vi "写入固件.vi"(8 "错误输入":errorcluster, 11 "MB session in":refnum<class "MB_Master.lvclass">) -> (0 "error out":errorcluster, 3 "MB session out":refnum<class "MB_Master.lvclass">)   [LabVIEW 2016, in "斯坦道氨氮.lvlib"]
uses:
  <vilib>/Plasmionique/MB Master/MB_Master/MB_Master.lvclass
  <vilib>/NI/Progress Bar/Controls/Update Bar Actions.ctl
  <vilib>/NI/Progress Bar/Controls/Progress Bar Properties.ctl
  <vilib>/Plasmionique/MB Master/MB_Master_Serial/MB_Master_Serial.lvclass
  C:/Program Files (x86)/National Instruments/LabVIEW 2016/vi.lib/Plasmionique/MB Master/MB_Master/MB_Master.lvclass
  <vilib>/Plasmionique/MB Master/MB Master.lvlib
  <vilib>/NI/Progress Bar/Progress Bar.lvlib
panel:
  in  "引用选择":enum16{"MB引用", "自建引用"}(ring)
  in  "VISA Resource":refnum<visa-resource-name>
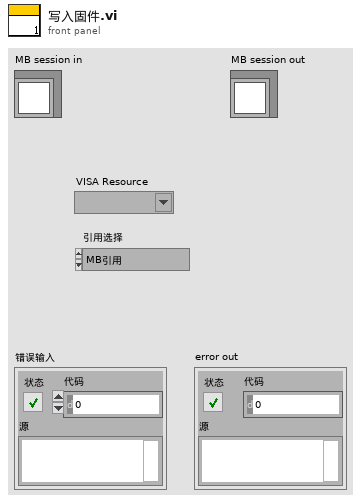
[diagram p1: front panel]
types:
  T1 = enum16{"open", "replace", "create", "open or create", "replace or create", "replace or create with confirmation"}
  T2 = enum16{"big-endian, network order", "native, host order", "little-endian"}
  T3 = typedef "Progress Bar.lvlib/Update Bar Actions.ctl" = enum16{"Add To Existing", "Set to Value"}
  T4 = cluster{"baud rate (bps)":u32, "stop bits":u16, "parity":u16, "flow control":u16, "timeout":u32, "retries":i32}
  T5 = typedef "Progress Bar.lvlib/Progress Bar Properties.ctl" = cluster{"Background Color":u32, "Installer Title":string, "Title Color":u32, "Action Text":string, "Text Color":u32, "Slider Value":u8, "Bar Color":u32, "Timeout":i32}
  T6 = cluster{"泵类型":u8, "进样速度":u32, "出样速度":u32, "泵阀量":u8, "光谱仪类型":u8, "光谱采样次数":u8, "氙灯次数":u8, "B":u16, "C":u16, "D":u16, "E":u16, "B_COD":u16, "C_COD":u16, "D_COD":u16, "E_COD":u16, "G":u16, "M":u16, "N":u16, "氨氮注射泵控温下限":sgl, "氨氮注射泵控温上限":sgl, "总氮注射泵控温下限":sgl, "总氮注射泵控温上限":sgl, "消解温度下限":sgl, "消解温度上限":sgl, "加热10s限值":sgl, "高温高压阀开阀温度":sgl, "总氮x公式0":u8, "总氮x公式1":sgl, "总氮x公式2":sgl, "总磷浊度稀释系数":sgl, "总磷浊度补偿权重1":sgl, "总磷浊度补偿权重2":sgl, "盐度系数":sgl, "氨氮补偿系数1":sgl, "氨氮补偿系数2":sgl}
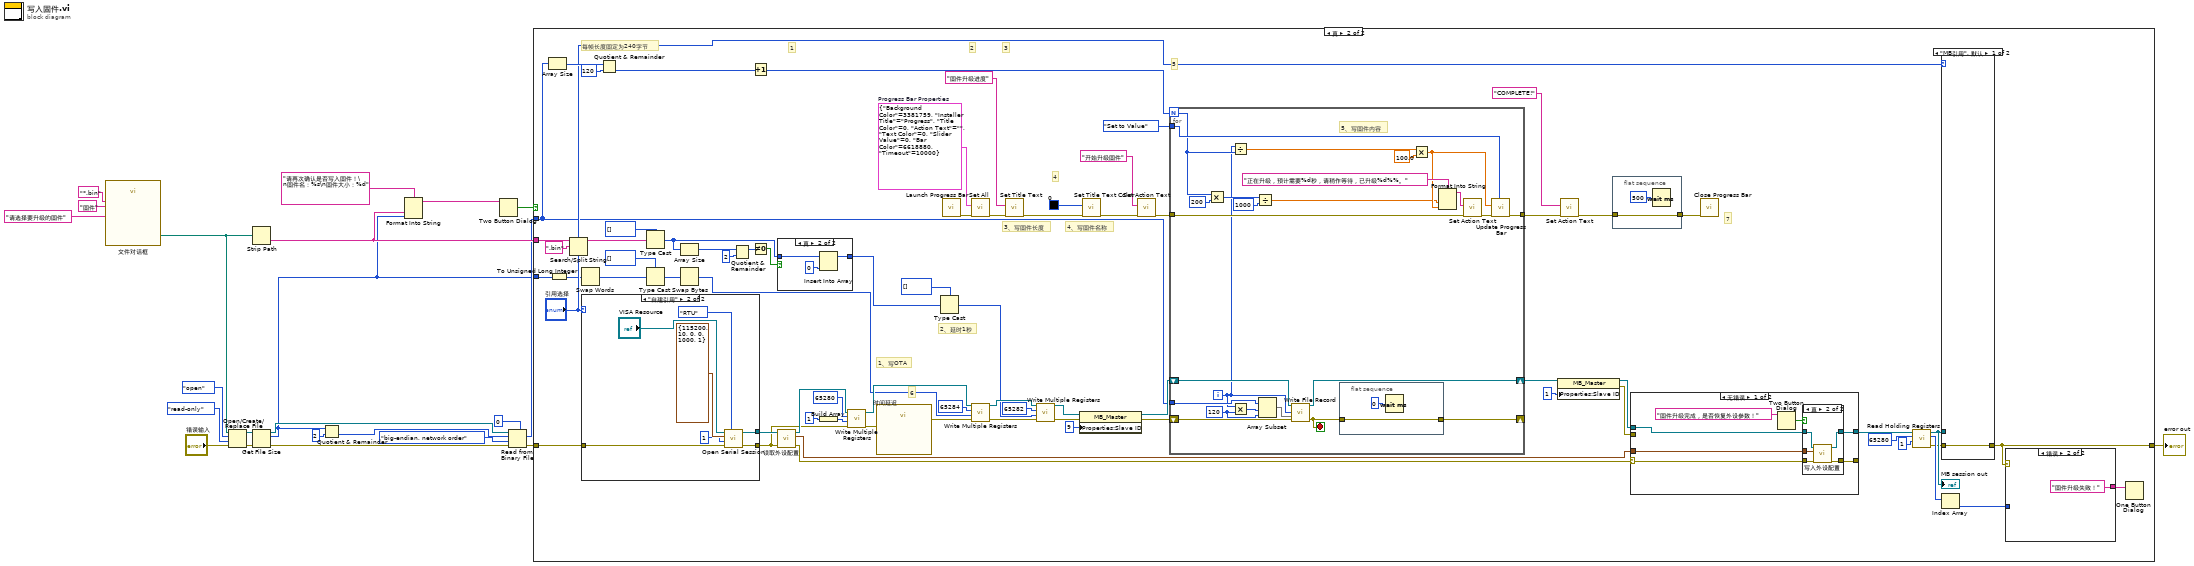
[diagram p0: block diagram]
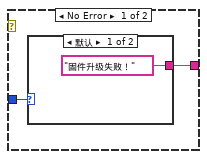
[diagram p6: hidden frame]
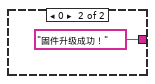
[diagram p7: hidden frame]
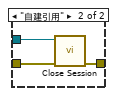
[diagram p8: hidden frame]
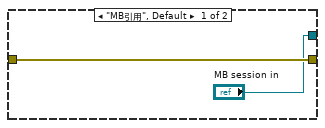
[diagram p9: hidden frame]
diagram:
  n1 = call "文件对话框"("prompt"="请选择要升级的固件", "pattern (all files)"="*.bin", "pattern label"="固件") -> ("selected path"=w10:path)  [unwired: 9 in, 3 out]
  n2 = Open/Create/Replace File(file path (use dialog)=w10, error in="错误输入", operation (0:open)=T1."open" ("操作(0:open)"), access (0:read/write)=enum16{"read/write", "read-only", "write-only"}."read-only" ("权限(0:read/write)")) -> (refnum out=w9:refnum<file>, error out=w7:errorcluster)  [unwired: 2 in, 1 out]
  n3 = Strip Path(path=w10) -> (name=w18:string)  [unwired: 1 out]
  n4 = Get File Size(file=w9, error in=w7) -> (refnum out=w8:refnum<file>, size (in bytes)=w2:i64, 0:w6:errorcluster)
  n5 = Quotient & Remainder(x=w2, y=i64 2) -> (floor(x/y)=w4:i64)  [unwired: 1 out]
  n6 = Format Into String(format string="请再次确认是否写入固件！\n固件名：%s\n固件大小：%d" ("格式字符串"), w18, w2) -> (resulting string=w17:string)  [unwired: 2 in, 1 out]
  n7 = Two Button Dialog(message=w17) -> (T button?=w16:bool)  [unwired: 2 in]
  n8 = Read from Binary File(5:u16 0, 8:w6, 9:T2."big-endian, network order" ("字节顺序(0:big-endian, network order)"), 10:w4, 11:w8) -> (0:w15:errorcluster, 2:w3:u16[])  [unwired: 1 in, 2 out]
  n9 = case shown="真" w16 {
    tunnel: w3 -> [_ w28]
    tunnel: w18 -> [_ w81]
    tunnel: w15 -> [w24 w82]
    tunnel: [w24 w56] -> w13
    tunnel: w2 -> [_ w68]
    frame False {
    }
    frame True {
      w53 = T5 {"Background Color"=3381759, "Installer Title"="Progress", "Title Color"=0, "Action Text"="", "Text Color"=0, "Slider Value"=0, "Bar Color"=6618880, "Timeout"=10000}  # Progress Bar Properties
      # "7"
      # "6"
      # "5"
      # "4"
      # "3"
      # "2"
      # "1"
      # "每帧长度固定为240字节"
      # "4、写固件名称"
      # "3、写固件长度"
      # "2、延时1秒"
      # "1、写OTA"
      n10 = Array Size(array=w28) -> (size(s)=w96:i32)
      n11 = To Unsigned Long Integer(number=w68) -> (unsigned 32bit integer=w61:u32)
      n12 = Search/Split String(string=w81, search string/char (-)=".bin" ("搜索字符串/字符(-)")) -> (substring before match=w79:string)  [unwired: 1 in, 2 out]
      n13 = Swap Words(1:w61) -> (0:w60:u32)
      n14 = case shown="\"自建引用\"" "引用选择" {
        tunnel: ["MB session in" w135] -> w83
        tunnel: w82 -> [w129 w134]
        tunnel: [w129 w133] -> w37
        frame "MB引用", Default {
        }
        frame "自建引用" {
          n15 = call <vilib>:"Open Serial Session.vi"("Mode (RTU)"=enum16{"RTU", "ASCII"}."RTU", "Error in"=w134, "Slave ID"=u8 1, "Serial Config"=T4 {"baud rate (bps)"=115200, "stop bits"=10, "parity"=0, "flow control"=0, "timeout"=1000, "retries"=1}, "VISA Resource"="VISA Resource") -> ("Error out"=w133:errorcluster, "MB_Serial session"=w135:refnum<class "MB_Master_Serial.lvclass">)  [unwired: 5 in]
        }
      }
      n16 = Quotient & Remainder(x=w96, y=120) -> (floor(x/y)=w27:i32)  [unwired: 1 out]
      n17 = Type Cast(type=u16[] [], x=w60) -> (*(type *) &x=w90:u16[])
      n18 = Type Cast(type=u8[] [], x=w79) -> (*(type *) &x=w31:u8[])
      n19 = Array Size(array=w31) -> (size(s)=w35:i32)
      n20 = Swap Bytes(anything=w90) -> (byte swapped=w29:u16[])
      n21 = Quotient & Remainder(x=w35, y=2) -> (x-y*floor(x/y)=w33:i32)  [unwired: 1 out]
      n22 = Increment(x=w27) -> (x+1=w67:i32)
      n23 = Not Equal To 0?(x=w33) -> (x != 0?=w32:bool)
      n24 = case shown="真" w32 {
        tunnel: w31 -> [w97 w100]
        tunnel: [w97 w99] -> w30
        frame False {
        }
        frame True {
          n25 = Insert Into Array(array=w100, new element=u8 0 ("新元素/子数组")) -> (w99:u8[])  [unwired: 1 in]
        }
      }
      n26 = call "读取外设配置.vi"("error in (no error)"=w37, "MB session in"=w83) -> ("error out"=w26:errorcluster, "外设配置"=w36:T6, "MB session out"=w39:refnum<class "MB_Master.lvclass">)  [unwired: 7 in]
      n27 = Build Array(u16 1 ("value")) -> (w84:u16[])
      n28 = call <vilib>:"Write Multiple Registers.vi"("error in (no error)"=w37, "values"=w84, "starting address"=u16 65280, "MB session in"=w39) -> ("error out"=w92:errorcluster, "MB session out"=w71:refnum<class "MB_Master.lvclass">)  [unwired: 6 in]
      n29 = call "时间延迟"("error in (no error)"=w92) -> ("error out"=w72:errorcluster)  [unwired: 10 in]
      n30 = Type Cast(type=u16[] [], x=w30) -> (*(type *) &x=w78:u16[])
      n31 = call <vilib>:"Launch Progress Bar.vi"() -> ("error out"=w52:errorcluster)  [unwired: 10 in, 1 out]
      n32 = call <vilib>:"Set All.vi"("error in (no error)"=w52, "Progress Bar Properties (Default)"=w53) -> ("error out"=w46:errorcluster)  [unwired: 9 in]
      n33 = call <vilib>:"Write Multiple Registers.vi"("error in (no error)"=w72, "values"=w29, "starting address"=u16 65284, "MB session in"=w71) -> ("error out"=w88:errorcluster, "MB session out"=w89:refnum<class "MB_Master.lvclass">)  [unwired: 6 in]
      n34 = call <vilib>:"Set Title Text.vi"("error in (no error)"=w46, "Installer Title"="固件升级进度") -> ("error out"=w44:errorcluster)  [unwired: 9 in]
      n35 = call <vilib>:"Write Multiple Registers.vi"("error in (no error)"=w88, "values"=w78, "starting address"=u16 65282, "MB session in"=w89) -> ("error out"=w63:errorcluster, "MB session out"=w66:refnum<class "MB_Master.lvclass">)  [unwired: 6 in]
      n36 = property class="MB_Master"(reference=w66, error in=w63, "Properties:Slave ID"=u8 9 ("Slave ID")) -> (reference out=w64:refnum<class "MB_Master.lvclass">, error out=w62:errorcluster)
      n37 = call <vilib>:"Set Title Text Color.vi"("error in (no error)"=w44, "Color Box"=u32 0) -> ("error out"=w47:errorcluster)  [unwired: 9 in]
      n38 = call <vilib>:"Set Action Text.vi"("error in (no error)"=w47, "Action Text"="开始升级固件") -> ("error out"=w41:errorcluster)  [unwired: 9 in]
      n39 = for {
        N: w67 -> [w141]
        shift-right: [w158] -> w59
        shift-left: w64 -> [w160]
        shift-right: [w137] -> _
        shift-left: w62 -> [w159]
        tunnel: w28 -> [w156]
        tunnel: Update_Bar_Actions."Set to Value" ("Action") -> [w152]
        tunnel: w41 -> [w150]
        tunnel: [w151] -> w40
        i -> [w139]
        stop <- w138 stop-if-true
        w154 = 120 ("长度")
        # "5、写固件内容"
        n40 = Multiply(x=w141, y=200) -> (x*y=w145:i32)
        n41 = Divide(x=w139, y=w141) -> (x/y=w146:dbl)
        n42 = Multiply(x=w139, y=w154) -> (x*y=w153:i32)
        n43 = Divide(x=w145, y=u32 1000) -> (x/y=w142:dbl)
        n44 = Array Subset(array=w156, index=w153, length=w154) -> (w155:u16[])
        n45 = call "Write File Record.vi"("MB session in"=w160, "Record Number"=w139, "values"=w155, "error in (no error)"=w159) -> ("MB session out"=w158:refnum<class "MB_Master.lvclass">, "error out"=w138:errorcluster)  [unwired: 10 in]
        n46 = flat-sequence {
          tunnel: w138 -> [w162]
          tunnel: [w162] -> w137
          frame #0 {
            n47 = Wait (ms)(milliseconds to wait=u32 0 ("等待时间（毫秒）")) -> ()  [unwired: 1 out]
          }
        }
        n48 = Multiply(x=w146, y=100.0) -> (x*y=w143:dbl)
        n49 = Format Into String(format string="正在升级，预计需要%d秒，请稍作等待，已升级%d%%。" ("格式字符串"), w142, w143) -> (resulting string=w147:string)  [unwired: 2 in, 1 out]
        n50 = call <vilib>:"Set Action Text.vi"("error in (no error)"=w150, "Action Text"=w147) -> ("error out"=w149:errorcluster)  [unwired: 9 in]
        n51 = call <vilib>:"Update Progress Bar.vi"("Action"=w152, "error in (no error)"=w149, "Value"=w143) -> ("error out"=w151:errorcluster)  [unwired: 8 in]
      }
      n52 = property class="MB_Master"(reference=w59, "Properties:Slave ID"=u8 1 ("Slave ID")) -> (reference out=w58:refnum<class "MB_Master.lvclass">, error out=w25:errorcluster)  [unwired: 1 in]
      n53 = call <vilib>:"Set Action Text.vi"("error in (no error)"=w40, "Action Text"="COMPLETE!") -> ("error out"=w49:errorcluster)  [unwired: 9 in]
      n54 = flat-sequence {
        tunnel: w49 -> [w117]
        tunnel: [w117] -> w51
        frame #0 {
          n55 = Wait (ms)(milliseconds to wait=u32 500) -> ()  [unwired: 1 out]
        }
      }
      n56 = case shown="无错误" w26 {
        selector: w26 -> [w101 w115]
        tunnel: w58 -> [w107 w116]
        tunnel: [w106 w116] -> w38
        tunnel: [w105 w115] -> _
        tunnel: w36 -> [w104 _]
        tunnel: w25 -> [_ _]
        frame No Error {
          n57 = Two Button Dialog(message="固件升级完成，是否恢复外设参数！" ("消息")) -> (T button?=w102:bool)  [unwired: 2 in]
          n58 = case shown="真" w102 {
            tunnel: w107 -> [w109 w114]
            tunnel: [w109 w113] -> w106
            tunnel: w101 -> [w108 w112]
            tunnel: [w108 w111] -> w105
            tunnel: w104 -> [_ w110]
            frame False {
            }
            frame True {
              n59 = call "写入外设配置.vi"("error in (no error)"=w112, "外设配置"=w110, "MB session in"=w114) -> ("error out"=w111:errorcluster, "MB session out"=w113:refnum<class "MB_Master.lvclass">)  [unwired: 7 in]
            }
          }
        }
        frame Error {
        }
      }
      n60 = call <vilib>:"Close Progress Bar.vi"("error in (no error)"=w51) -> ()  [unwired: 9 in, 2 out]
      n61 = call <vilib>:"Read Holding Registers.vi"("quantity"=u16 1, "starting address"=u16 65280, "MB session in"=w38) -> ("error out"=w69:errorcluster, "Registers"=w73:u16[], "MB session out"=w70:refnum<class "MB_Master.lvclass">)  [unwired: 6 in]
      "MB session out" <- w70
      n62 = case shown="\"MB引用\", 默认" "引用选择" {
        tunnel: w70 -> [_ w127]
        tunnel: w69 -> [w124 w126]
        tunnel: [w124 w125] -> w56
        frame "MB引用", Default {
        }
        frame "自建引用" {
          n63 = call-dynamic "Close Session.vi"("error in (no error)"=w126, "MB session in"=w127) -> ("error out"=w125:errorcluster)  [unwired: 9 in]
        }
      }
      n64 = Index Array(array=w73) -> (element=w55:u16)  [unwired: 1 in]
      n65 = case shown="错误" w56 {
        tunnel: w55 -> [w120 _]
        tunnel: [w119 "固件升级失败！"] -> w54
        frame No Error {
          n66 = case shown="默认" w120 {
            tunnel: ["固件升级失败！" "固件升级成功！"] -> w119
            frame Default {
            }
            frame 0 {
            }
          }
        }
        frame Error {
        }
      }
      n67 = One Button Dialog(message=w54) -> ()  [unwired: 1 in, 1 out]
    }
  }
  "error out" <- w13
